vi "C1--d Hi.vi"(8 "Command Info In":T2, 10 "Corridor to Diag Scale":T1={"1t"=38.0, "2d"=55.0, "2s"=0.65, "3a"=6.0, "4d"=10.0, "4s"=0.5}, 11 "Scale":string) -> (0 "Command Info Out":T2)   [LabVIEW 2017]
uses:
  <vilib>/Rock Robotics/WPI/Framework/Command Status Info.ctl
  <vilib>/Rock Robotics/WPI/Framework/Completion Status.ctl
  <vilib>/Rock Robotics/WPI/Framework/Completion Notifier.ctl
  Block Clusters/C1--d Hi.ctl
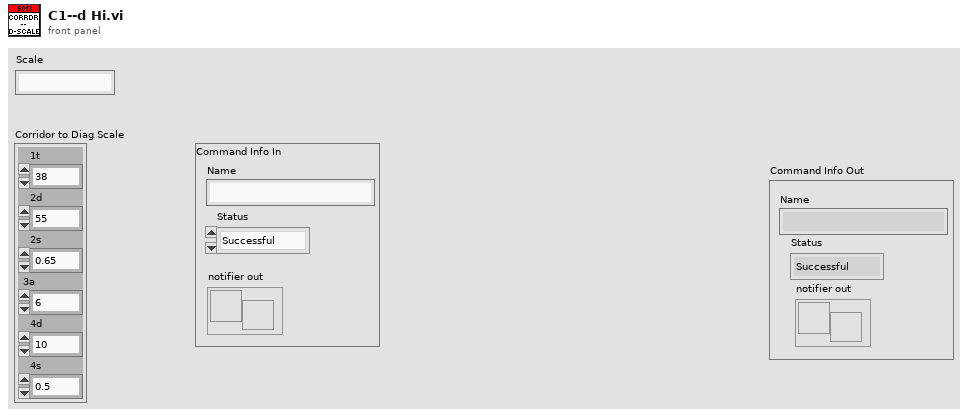
[diagram p1: front panel]
types:
  T1 = typedef "C1--d Hi.ctl" = cluster{"1t":dbl, "2d":dbl, "2s":dbl, "3a":dbl, "4d":dbl, "4s":dbl}
  T2 = typedef "Command Status Info.ctl" = cluster{"Name":string, "Status":T3, "notifier out":T4}
  T3 = typedef "Completion Status.ctl" = enum16{"Successful", "Aborted", "Incomplete"}
  T4 = typedef "Completion Notifier.ctl" = refnum<notifier>
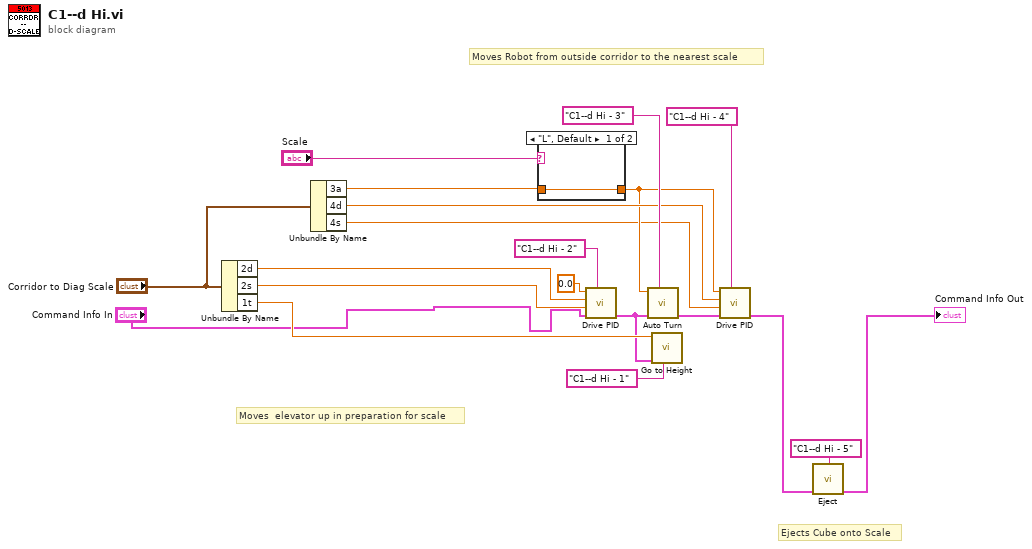
[diagram p0: block diagram]
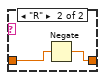
[diagram p2: hidden frame]
diagram:
  # "Moves  elevator up in preparation for scale"
  # "Ejects Cube onto Scale"
  # "Moves Robot from outside corridor to the nearest scale"
  n1 = Unbundle By Name("Corridor to Diag Scale") -> ("2d"=w20:dbl, "2s"=w19:dbl, "1t"=w18:dbl)
  n2 = Unbundle By Name("Corridor to Diag Scale") -> ("3a"=w10:dbl, "4d"=w6:dbl, "4s"=w4:dbl)
  n3 = case shown="\"L\", Default" "Scale" {
    tunnel: [w21 w23] -> w5
    tunnel: w10 -> [w21 w22]
    frame "L", Default {
    }
    frame "R" {
      n4 = Negate(x=w22) -> (-x=w23:dbl)
    }
  }
  n5 = call "Drive PID.vi"("Description"="C1--d Hi - 2", "Command Info In"="Command Info In", "Speed"=w19, "Distance"=w20, "Target Angle"=0.0) -> ("Command Info Out"=w1:T2)  [unwired: 6 in]
  n6 = call "Auto Turn.vi"("Description"="C1--d Hi - 3", "Command Info In"=w1, "Target Angle"=w5) -> ("Command Info Out"=w8:T2)  [unwired: 8 in]
  n7 = call "Go to Height.vi"("Description"="C1--d Hi - 1", "Command Info In"=w1, "Target Height (in)"=w18) -> ()  [unwired: 8 in, 1 out]
  n8 = call "Drive PID.vi"("Description"="C1--d Hi - 4", "Command Info In"=w8, "Speed"=w4, "Distance"=w6, "Target Angle"=w5) -> ("Command Info Out"=w3:T2)  [unwired: 6 in]
  n9 = call "Eject.vi"("Description"="C1--d Hi - 5", "Command Info In"=w3) -> ("Command Info Out"=→"Command Info Out":T2)  [unwired: 9 in]
